vi "lockin.vi"() -> ()   [LabVIEW 2012]
panel:
  out "Numeric":dbl
  out "Lockin X (V)":dbl=0.000877265
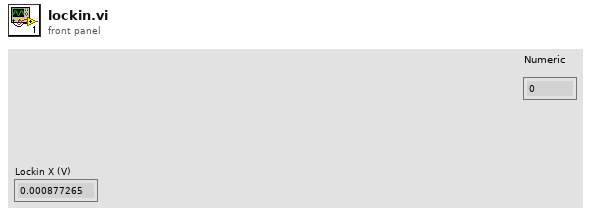
[diagram p1: front panel]
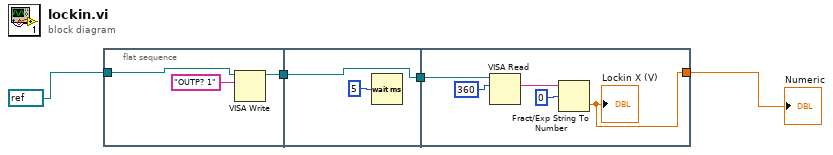
[diagram p0: block diagram]
diagram:
  n1 = flat-sequence {
    tunnel: refnum<visa-resource-name> "GPIB0::8::INSTR" ("Lockin SR830") -> [w7]
    tunnel: [w5] -> w4
    tunnel: [w8] -> w3
    tunnel: w4 -> [w8]
    tunnel: w3 -> [w12]
    tunnel: [w10] -> w1
    frame #0 {
      n2 = VISA Write(VISA resource name=w7, write buffer="OUTP? 1" ("write buffer 2")) -> (VISA resource name out=w5:refnum<visa-resource-name>)  [unwired: 1 in, 2 out]
    }
    frame #1 {
      n3 = Wait (ms)(milliseconds to wait=5) -> ()  [unwired: 1 out]
    }
    frame #2 {
      n4 = VISA Read(VISA resource name=w12, byte count=u32 360) -> (read buffer=w11:string)  [unwired: 1 in, 3 out]
      n5 = Fract/Exp String To Number(string=w11, offset=0) -> (number=w10:dbl)  [unwired: 3 out]
      "Lockin X (V)" <- w10
    }
  }
  "Numeric" <- w1
